vi "InitApp.vi"() -> ()   [LabVIEW 2013]
panel:
  out "error out":errorcluster
  in  "error in":errorcluster
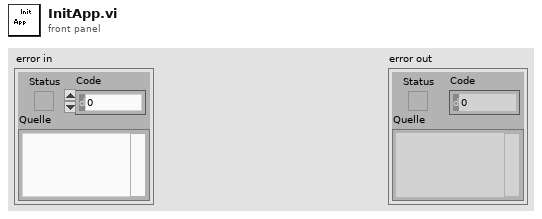
[diagram p1: front panel]
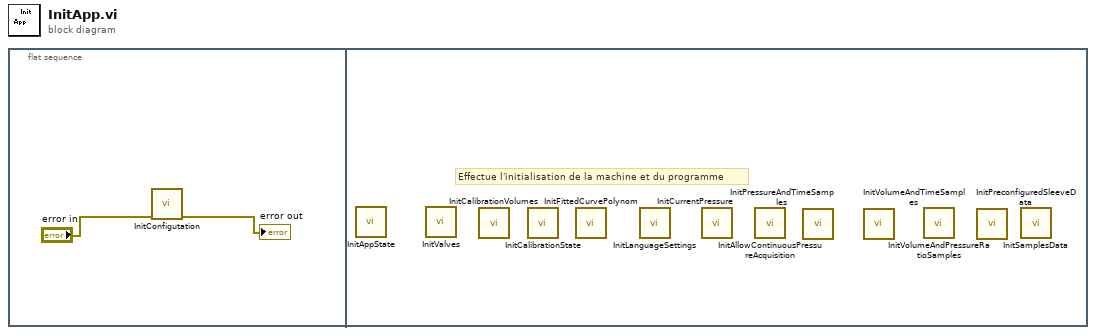
[diagram p0: block diagram]
diagram:
  n1 = flat-sequence {
    frame #0 {
      n2 = call "InitConfigutation.vi"("error in"="error in") -> ("error out"=→"error out":errorcluster)  [unwired: 10 in]
    }
    frame #1 {
      # "Effectue l'initialisation de la machine et du programme"
      n3 = call "InitAppState.vi"() -> ()  [unwired: 12 in]
      n4 = call "InitValves.vi"() -> ()  [unwired: 12 in]
      n5 = call "InitCalibrationVolumes.vi"() -> ()  [unwired: 12 in]
      n6 = call "InitCalibrationState.vi"() -> ()  [unwired: 12 in]
      n7 = call "InitFittedCurvePolynom.vi"() -> ()  [unwired: 12 in]
      n8 = call "InitLanguageSettings.vi"() -> ()  [unwired: 12 in]
      n9 = call "InitCurrentPressure.vi"() -> ()  [unwired: 12 in]
      n10 = call "InitAllowContinuousPressureAcquisition.vi"() -> ()  [unwired: 12 in]
      n11 = call "InitPressureAndTimeSamples.vi"() -> ()  [unwired: 12 in]
      n12 = call "InitVolumeAndTimeSamples.vi"() -> ()  [unwired: 12 in]
      n13 = call "InitVolumeAndPressureRatioSamples.vi"() -> ()  [unwired: 12 in]
      n14 = call "InitPreconfiguredSleeveData.vi"() -> ()  [unwired: 11 in, 1 out]
      n15 = call "InitSamplesData.vi"() -> ()  [unwired: 12 in]
    }
  }
